vi "VS-Read All.vi"(0 "Hardware Mutex":T1, 5 "Options":T2={"Min Interval"=0.0, "HR from ABR?"=FALSE, "HR Scale"={"Slope"=0.0, "Offset"=0.0, "Limits"={"Min"=0.0, "Max"=0.0}, "term config"=-1}, "Temp Scale"={"Slope"=0.0, "Offset"=0.0, "Limits"={"Min"=0.0, "Max"=0.0}, "term config"=-1}, "Lock?"=FALSE, "Temp Sensor"=enum."YSI", "EKG"={"Sample duration (s)"=0.0}} {"Temp Scale"."term config" items=["default"=-1, "RSE"=10083, "NRSE"=10078, "Differential"=10106, "Pseudodifferential"=12529]; "HR Scale"."term config" items=["default"=-1, "RSE"=10083, "NRSE"=10078, "Differential"=10106, "Pseudodifferential"=12529]}, 11 "error in (no error)":errorcluster) -> (4 "Timestamp":timestamp, 6 "Heart Rate (bpm)":dbl, 8 "Temperature (C)":dbl, 15 "error out":errorcluster)   [LabVIEW 2020]
uses:
  Typedefs/PhysMon-Options.ctl
  Typedefs/PhysMon-Scale.ctl
  Typedefs/PhysMon-TempSensor.ctl
  Typedefs/PhysMon-HR From EKG Settings.ctl
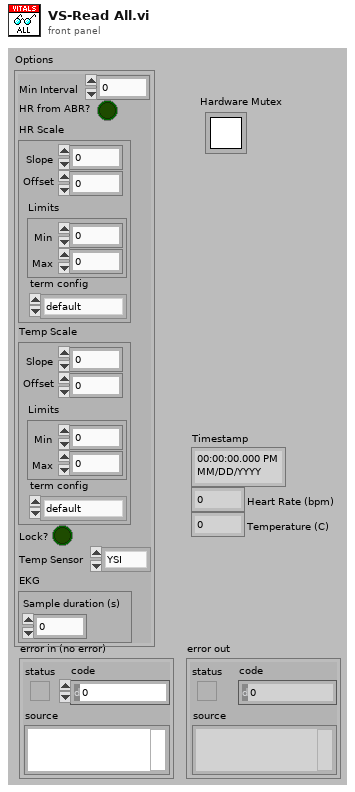
[diagram p1: front panel]
types:
  T1 = typedef "Semaphore RefNum" = refnum<k1>
  T2 = typedef "PhysMon-Options.ctl" = cluster{"Min Interval":dbl, "HR from ABR?":bool, "HR Scale":T3, "Temp Scale":T3, "Lock?":bool, "Temp Sensor":T4, "EKG":T5}
  T3 = typedef "PhysMon-Scale.ctl" = cluster{"Slope":dbl, "Offset":dbl, "Limits":cluster{"Min":dbl, "Max":dbl}, "term config":i32}
  T4 = typedef "PhysMon-TempSensor.ctl" = enum16{"YSI", "FHC", "Custom"}
  T5 = typedef "PhysMon-HR From EKG Settings.ctl" = cluster{"Sample duration (s)":dbl}
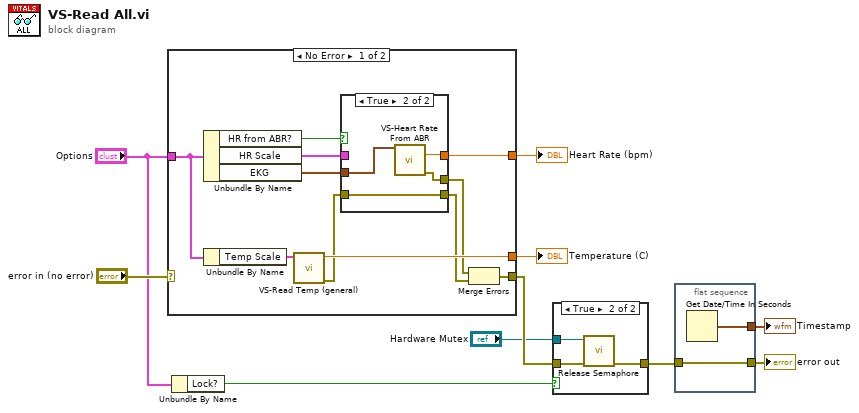
[diagram p0: block diagram]
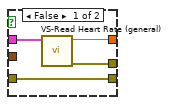
[diagram p3: hidden frame]
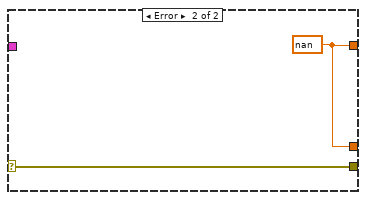
[diagram p4: hidden frame]
diagram:
  n1 = case shown="No Error" "error in (no error)" {
    selector: "error in (no error)" -> [_ w30]
    tunnel: [w15 w30] -> w7
    tunnel: [w21 w31] -> w4
    tunnel: "Options" -> [w18 _]
    tunnel: [w16 w31] -> w3
    frame No Error {
      n2 = Unbundle By Name(w18) -> ("HR from ABR?"=w20:bool, "HR Scale"=w19:T3, "EKG"=w11:T5)
      n3 = Unbundle By Name(w18) -> ("Temp Scale"=w17:T3)
      n4 = call "VS-Read Temp (general).vi"("Scale"=w17) -> ("error out"=w13:errorcluster, "Temp (C)"=w16:dbl)  [unwired: 8 in, 1 out]
      n5 = case shown="True" w20 {
        tunnel: [w25 w29] -> w21
        tunnel: w19 -> [w24 _]
        tunnel: [w23 w28] -> w14
        tunnel: w13 -> [w22 w27]
        tunnel: [w22 w27] -> w12
        tunnel: w11 -> [_ w26]
        frame False {
          n6 = call "VS-Read Heart Rate (general).vi"("Scale"=w24) -> ("error out"=w23:errorcluster, "Heart Rate (bpm)"=w25:dbl)  [unwired: 9 in]
        }
        frame True {
          n7 = call "VS-Heart Rate From ABR.vi"("Settings"=w26) -> ("Heart Rate (bpm)"=w29:dbl, "error out"=w28:errorcluster)  [unwired: 11 in, 2 out]
        }
      }
      n8 = Merge Errors(w14, w12) -> (w15:errorcluster)
    }
    frame Error {
      w31 = nan ("Heart Rate (bpm)")
    }
  }
  "Temperature (C)" <- w3
  "Heart Rate (bpm)" <- w4
  n9 = Unbundle By Name("Options") -> ("Lock?"=w1:bool)
  n10 = case shown="True" w1 {
    tunnel: w7 -> [w32 w35]
    tunnel: [w32 w34] -> w6
    tunnel: "Hardware Mutex" -> [_ w33]
    frame False {
    }
    frame True {
      n11 = call <vilib>:"Release Semaphore.vi"("error in (no error)"=w35, "semaphore"=w33) -> ("error out"=w34:errorcluster)  [unwired: 4 in, 1 out]
    }
  }
  n12 = flat-sequence {
    tunnel: w6 -> [w36]
    tunnel: [w36] -> w9
    tunnel: [w37] -> w8
    frame #0 {
      n13 = Get Date/Time In Seconds() -> (seconds since 1Jan1904=w37:timestamp)
    }
  }
  "error out" <- w9
  "Timestamp" <- w8
